vi "Waveform Samples.vi"(8 "error in (no error)":errorcluster {"code" format="%.0x"}, 10 "Trace Number (0: Scope Trace or Record)":i32(ring) items=["Scope Trace or Record", "Trend Plot", "Persistence", "Reference Trace", "Spectrum"], 11 "VISA resource name":refnum<visa-resource-name>) -> (0 "error out":errorcluster {"code" format="%.0x"}, 1 "Waveform Sample Information":T2 {"Sample Pairing" items=["Normal"=0, "Min/Max"=1, "Min/Max/Avg"=2, "Min=Max"=3, "Min=Max=Avg"=4, "Unknown Format"=7]; "Sample Format" items=["Unsigned", "Signed"]}, 2 "Waveform Amplitude":T1, 3 "VISA resource name out":refnum<visa-resource-name>)   [LabVIEW 2014, in "Fluke 190 Series II.lvlib"]
doc: "Formats the waveform samples and the waveform sample information needed in Read Waveform."
uses:
  Fluke 190 Series II.lvlib
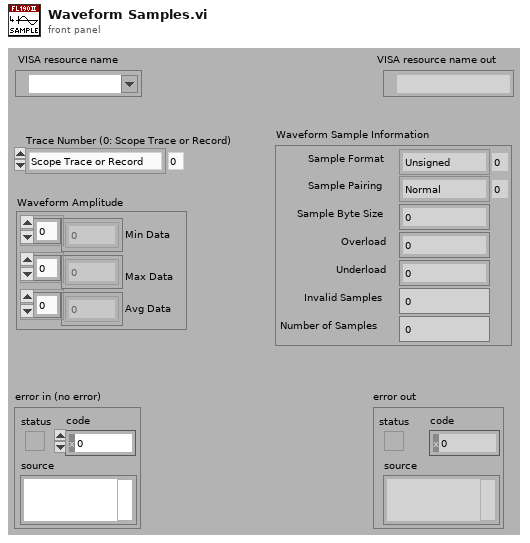
[diagram p1: front panel]
types:
  T1 = cluster{"Min Data":dbl[], "Max Data":dbl[], "Avg Data":dbl[]}
  T2 = cluster{"Sample Format":i16, "Sample Pairing":u8, "Sample Byte Size":u8, "Overload":dbl, "Underload":dbl, "Invalid Samples":dbl, "Number of Samples":u16}
  T3 = cluster{i16, "f":u8, u8, "Converted Output":dbl, "Converted Output":dbl, "Converted Output":dbl, u16}
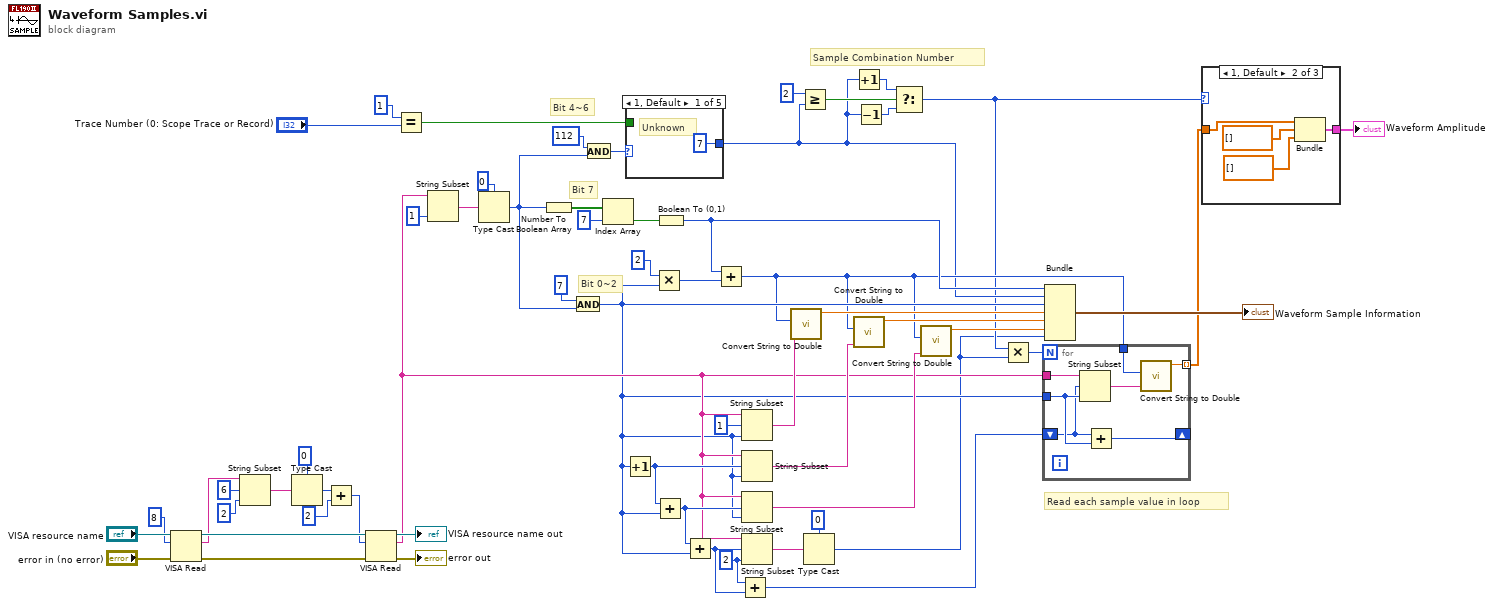
[diagram p0: block diagram]
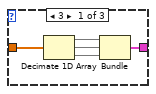
[diagram p2: hidden frame]
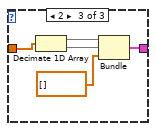
[diagram p3: hidden frame]
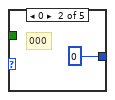
[diagram p4: hidden frame]
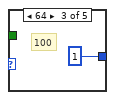
[diagram p5: hidden frame]
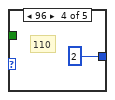
[diagram p6: hidden frame]
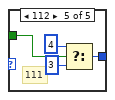
[diagram p7: hidden frame]
diagram:
  w20 = 2 ("length (rest)")
  # "Sample Combination Number"
  # "Read each sample value in loop"
  # "Bit 7"
  # "Bit 4~6"
  # "Bit 0~2"
  n1 = VISA Read(VISA resource name="VISA resource name", byte count=u32 8, error in (no error)="error in (no error)") -> (VISA resource name out=w56:refnum<visa-resource-name>, read buffer=w46:string, error out=w57:errorcluster)  [unwired: 1 out]
  n2 = String Subset(string=w46, offset (0)=6, length (rest)=2 ("length (rest)")) -> (substring=w50:string)
  n3 = Type Cast(type=u16 0 ("length (rest)"), x=w50) -> (*(type *) &x=w48:u16)
  n4 = Add(x=w48, y=u16 2) -> (x+y=w45:u16)
  n5 = VISA Read(VISA resource name=w56, byte count=w45, error in (no error)=w57) -> (VISA resource name out=→"VISA resource name out":refnum<visa-resource-name>, read buffer=w17:string, error out=→"error out":errorcluster)  [unwired: 1 out]
  n6 = Equal?(x=1, y="Trace Number (0: Scope Trace or Record)") -> (x = y?=w11:bool)
  n7 = String Subset(string=w17, length (rest)=1 ("length (rest)")) -> (substring=w42:string)  [unwired: 1 out]
  n8 = Type Cast(type=u8 0, x=w42) -> (*(type *) &x=w41:u8)
  n9 = Number To Boolean Array(number=w41) -> (Boolean array=w37:bool[])
  n10 = And(x=u8 7, y=w41) -> (x .and. y?=w16:u8)
  n11 = And(x=u8 112, y=w41) -> (x .and. y?=w40:u8)
  n12 = Index Array(array=w37, index=7) -> (element=w39:bool)
  n13 = Increment(x=w16) -> (x+1=w28:u8)
  n14 = case shown="1, Default" w40 {
    tunnel: [u8 7 u8 0 u8 1 u8 2 w64] -> w7
    tunnel: w11 -> [_ _ _ _ w67]
    frame 1, Default {
      # "Unknown"
    }
    frame 0 {
      # "000"
    }
    frame 64 {
      # "100"
    }
    frame 96 {
      # "110"
    }
    frame 112 {
      # "111"
      n15 = Select(t=u8 4, s=w67, f=u8 3) -> (s? t:f=w64:u8)
    }
  }
  n16 = Multiply(x=u8 2, y=w16) -> (x*y=w29:u8)
  n17 = Add(x=w28, y=w16) -> (x+y=w23:u8)
  n18 = Boolean To (0,1)(Boolean=w39) -> (0, 1=w30:i16)
  n19 = Add(x=w23, y=w16) -> (x+y=w19:u8)
  n20 = Add(x=w30, y=w29) -> (x+y=w14:i16)
  n21 = Add(x=w20, y=w19) -> (x+y=w15:i32)
  n22 = String Subset(string=w17, offset (0)=1, length (rest)=w16) -> (substring=w32:string)
  n23 = String Subset(string=w17, offset (0)=w28, length (rest)=w16) -> (substring=w26:string)
  n24 = String Subset(string=w17, offset (0)=w23, length (rest)=w16) -> (substring=w25:string)
  n25 = String Subset(string=w17, offset (0)=w19, length (rest)=w20) -> (substring=w22:string)
  n26 = call "Convert String to Double.vi"("Input String"=w32, "Conversion Type (6)"=w14) -> ("Converted Output"=w34:dbl)  [unwired: 1 in, 8 out]
  n27 = Greater Or Equal?(x=u8 2 ("y"), y=w7) -> (x >= y?=w10:bool)
  n28 = Type Cast(type=u16 0, x=w22) -> (*(type *) &x=w1:u16)
  n29 = Increment(x=w7) -> (x+1=w8:u8)
  n30 = call "Convert String to Double.vi"("Input String"=w26, "Conversion Type (6)"=w14) -> ("Converted Output"=w27:dbl)  [unwired: 1 in, 8 out]
  n31 = Decrement(x=w7) -> (x-1=w6:u8)
  n32 = Select(t=w8, s=w10, f=w6) -> (s? t:f=w2:u8)
  n33 = call "Convert String to Double.vi"("Input String"=w25, "Conversion Type (6)"=w14) -> ("Converted Output"=w24:dbl)  [unwired: 1 in, 8 out]
  n34 = Multiply(x=w2, y=w1) -> (x*y=w3:u16)
  n35 = for {
    N: w3 -> [_]
    tunnel: w17 -> [w74]
    tunnel: w16 -> [w73]
    shift-right: [w72] -> _
    shift-left: w15 -> [w71]
    tunnel: w14 -> [w69]
    tunnel: [w68] -> w5 mode=indexing
    n36 = String Subset(string=w74, offset (0)=w71, length (rest)=w73) -> (substring=w70:string)
    n37 = Add(x=w71, y=w73) -> (x+y=w72:i32)
    n38 = call "Convert String to Double.vi"("Input String"=w70, "Conversion Type (6)"=w69) -> ("Converted Output"=w68:dbl)  [unwired: 1 in, 8 out]
  }
  n39 = Bundle(w30, "f"=w7, w16, "Converted Output"=w34, "Converted Output"=w27, "Converted Output"=w24, w1) -> (→"Waveform Sample Information":T3)  [unwired: 1 out]
  n40 = case shown="1, Default" w2 {
    tunnel: w5 -> [w79 w83 w88]
    tunnel: [w75 w81 w84] -> w4
    frame 3 {
      n41 = Decimate 1D Array(w79) -> (w78:dbl[], w77:dbl[], w76:dbl[])
      n42 = Bundle(w78, w77, w76) -> (w75:cluster{dbl[], dbl[], dbl[]})  [unwired: 1 out]
    }
    frame 1, Default {
      n43 = Bundle(w83, dbl[] [], dbl[] []) -> (w81:cluster{dbl[], dbl[], dbl[]})  [unwired: 1 out]
    }
    frame 2 {
      n44 = Decimate 1D Array(w88) -> (w87:dbl[], w86:dbl[])
      n45 = Bundle(w87, w86, dbl[] []) -> (w84:cluster{dbl[], dbl[], dbl[]})  [unwired: 1 out]
    }
  }
  "Waveform Amplitude" <- w4
